vi "Run.vi"(8 "error in (no error)":errorcluster, 11 "Opctics in":refnum<class "Optics.lvclass">) -> (0 "error out":errorcluster, 3 "Optics out":refnum<class "Optics.lvclass">)   [LabVIEW 2018, in "Optics.lvclass"]
uses:
  Optics.lvclass
  Optics.lvclass/Optics.ctl
  Device.lvclass
  StateMachine/State Machine.lvclass
panel:
  out "on target 3":bool
  out "on target 2":bool
  out "on target":bool
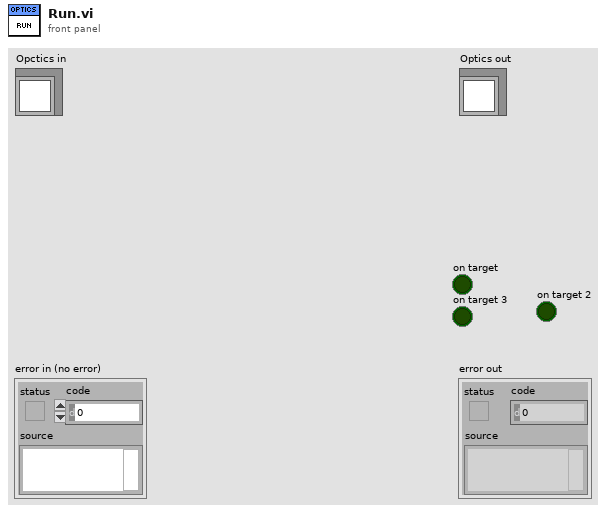
[diagram p1: front panel]
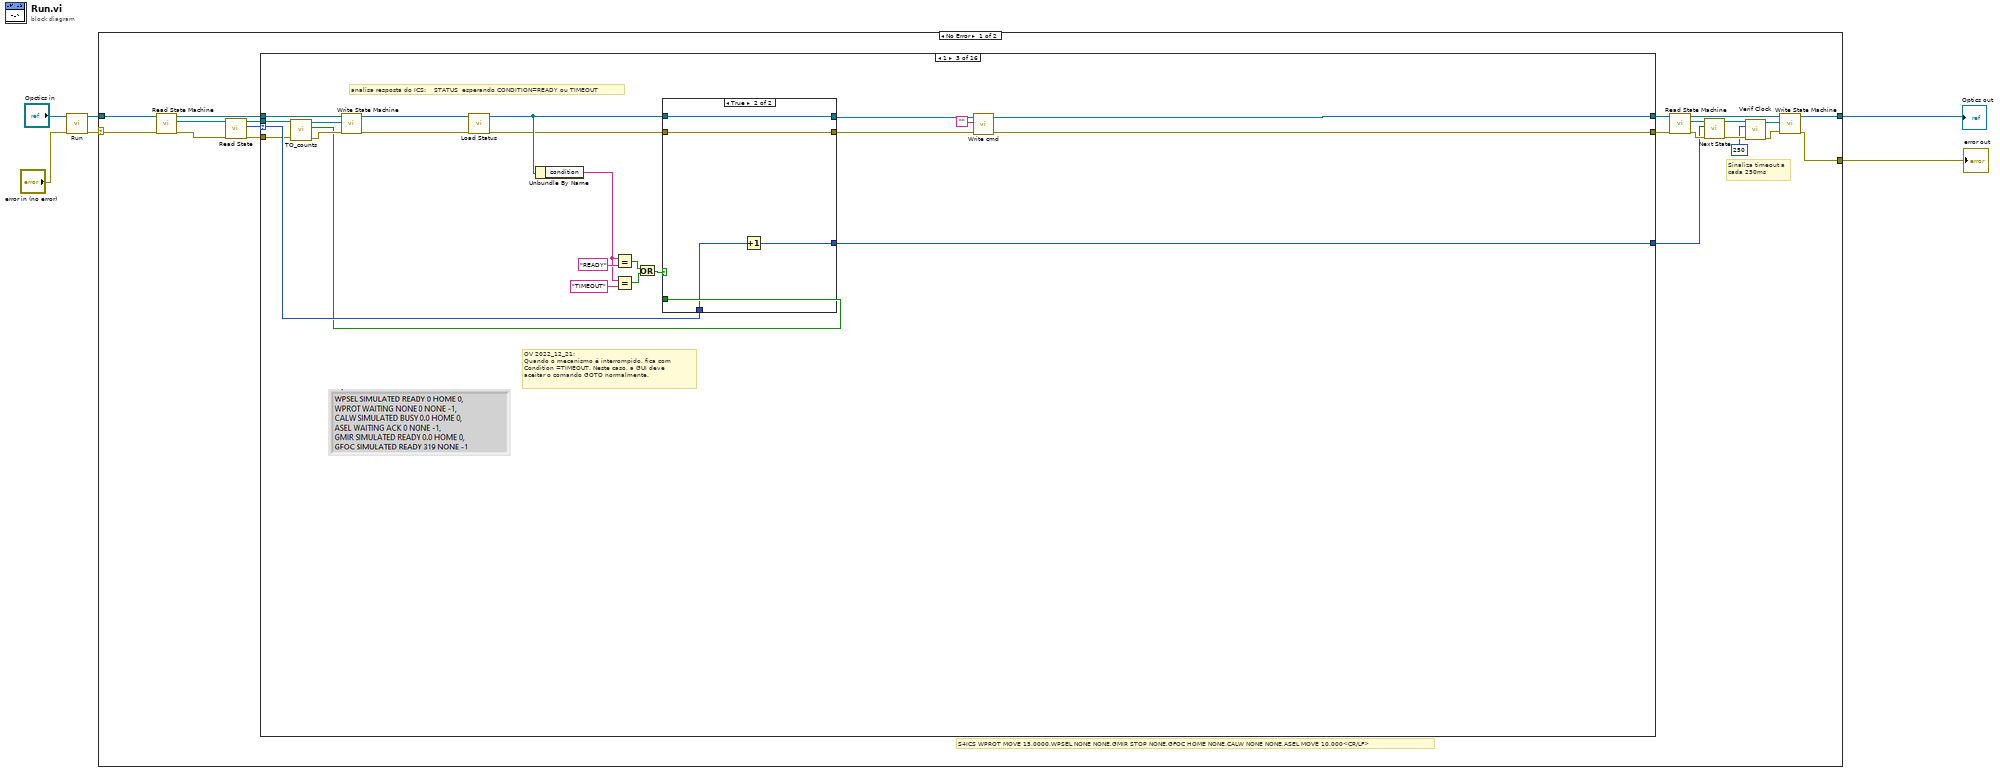
[diagram p0: block diagram]
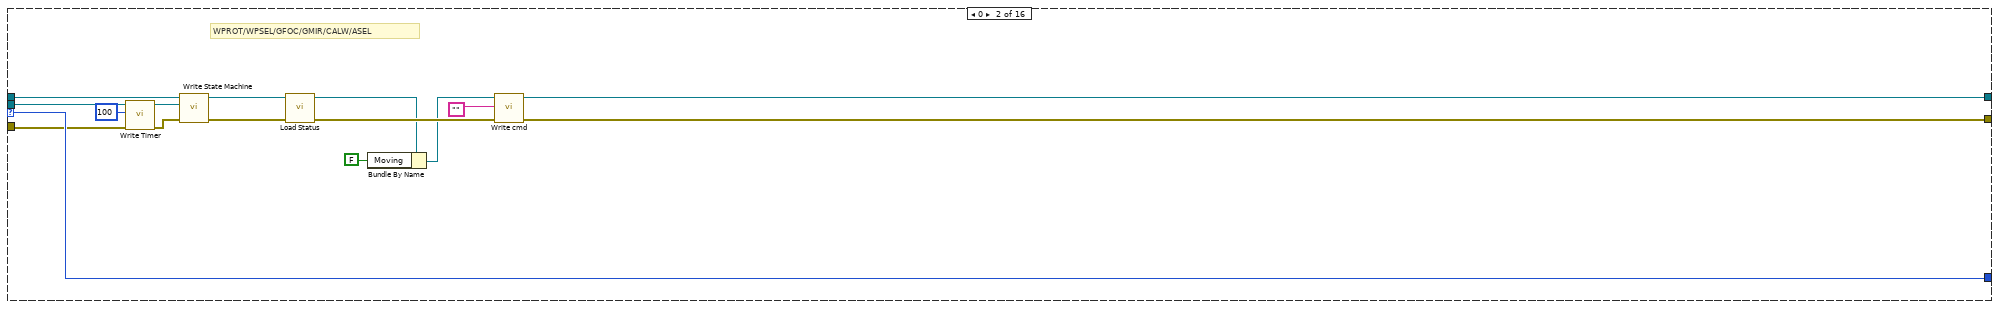
[diagram p3: hidden frame]
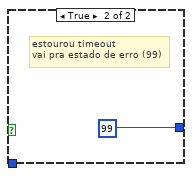
[diagram p5: hidden frame]
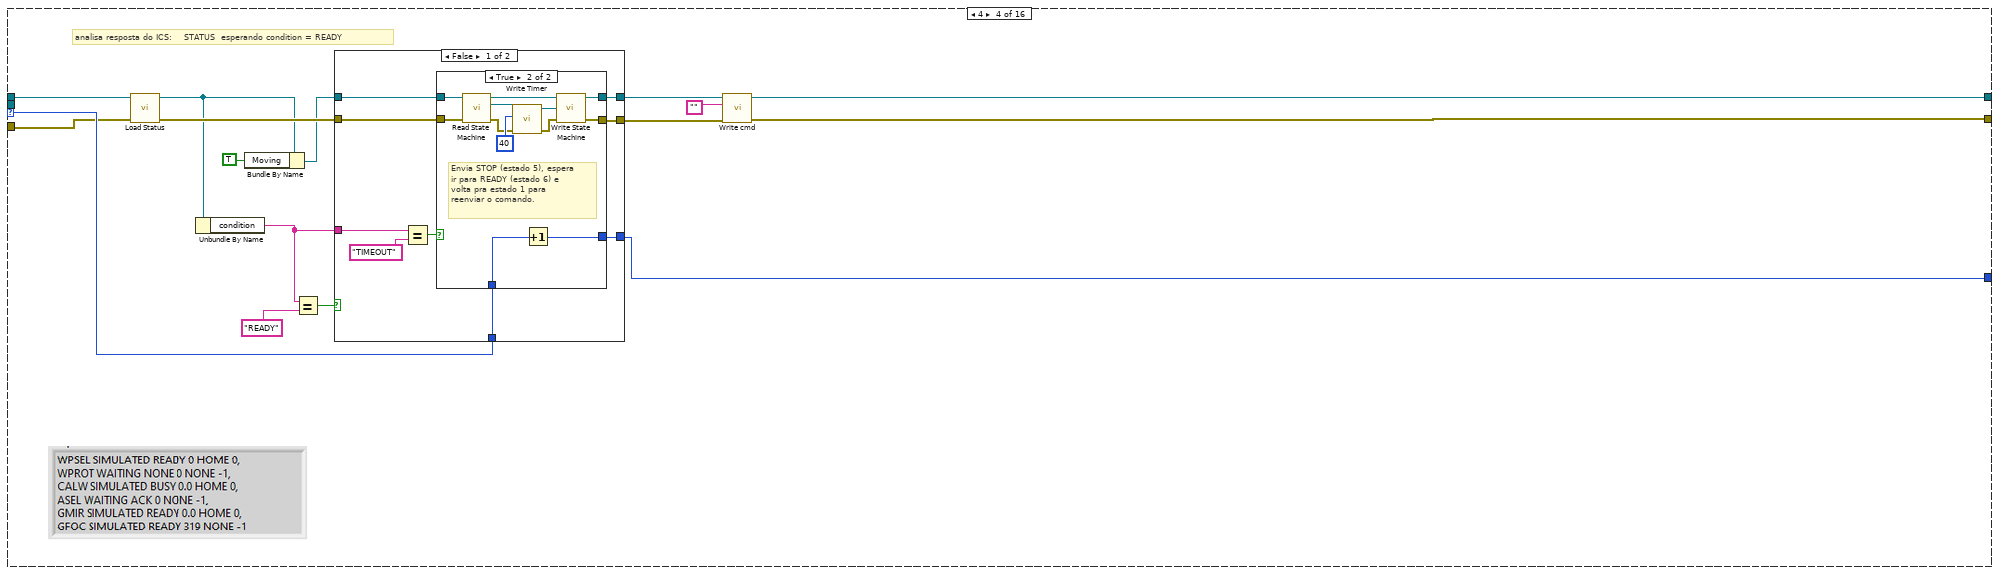
[diagram p6: hidden frame]
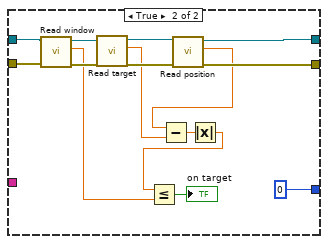
[diagram p8: hidden frame]
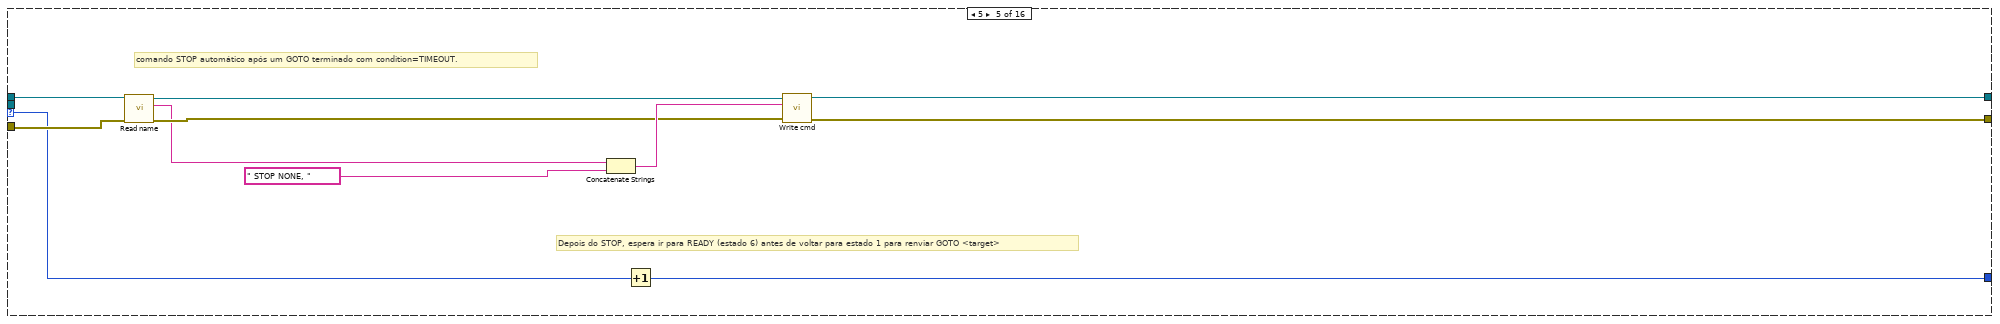
[diagram p9: hidden frame]
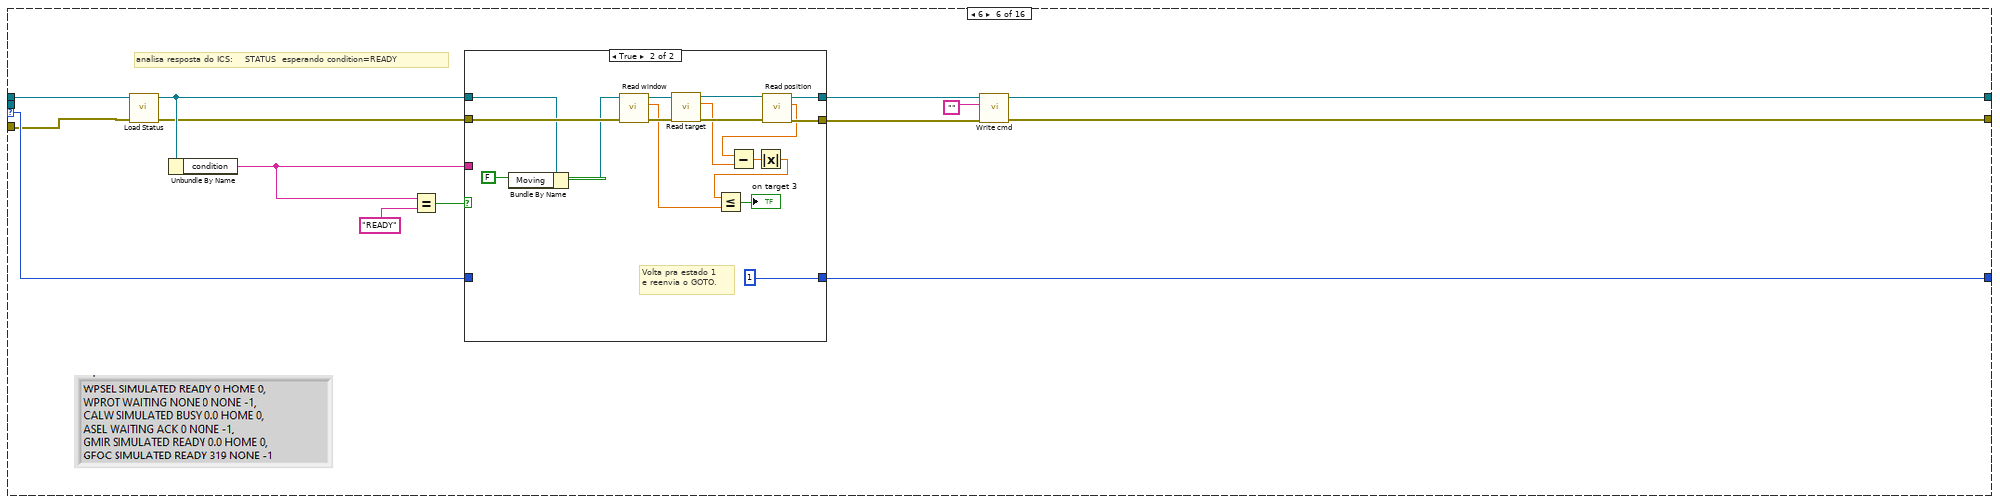
[diagram p10: hidden frame]
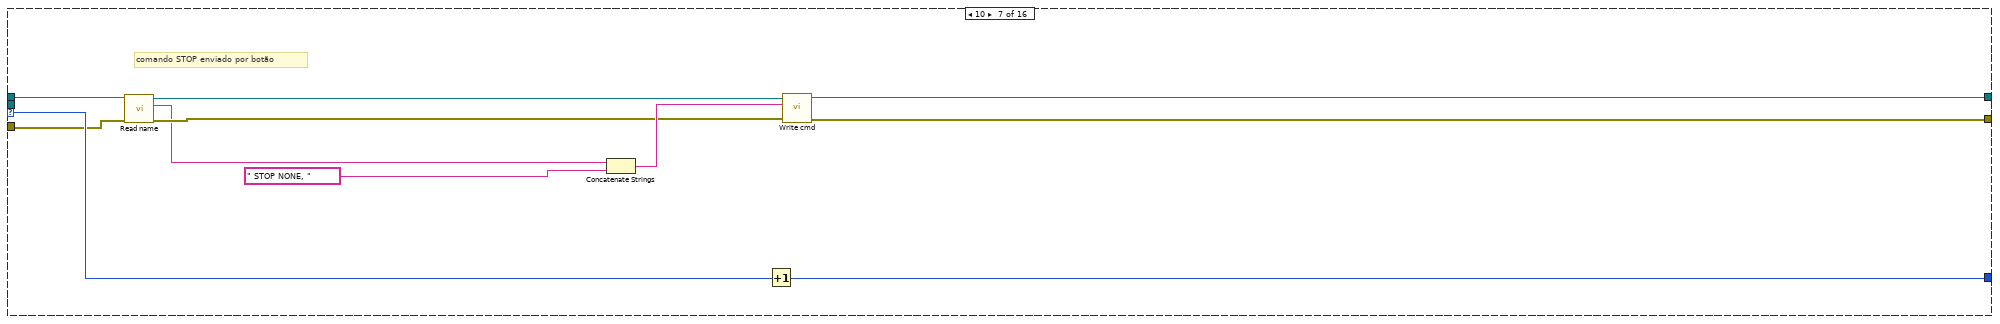
[diagram p12: hidden frame]
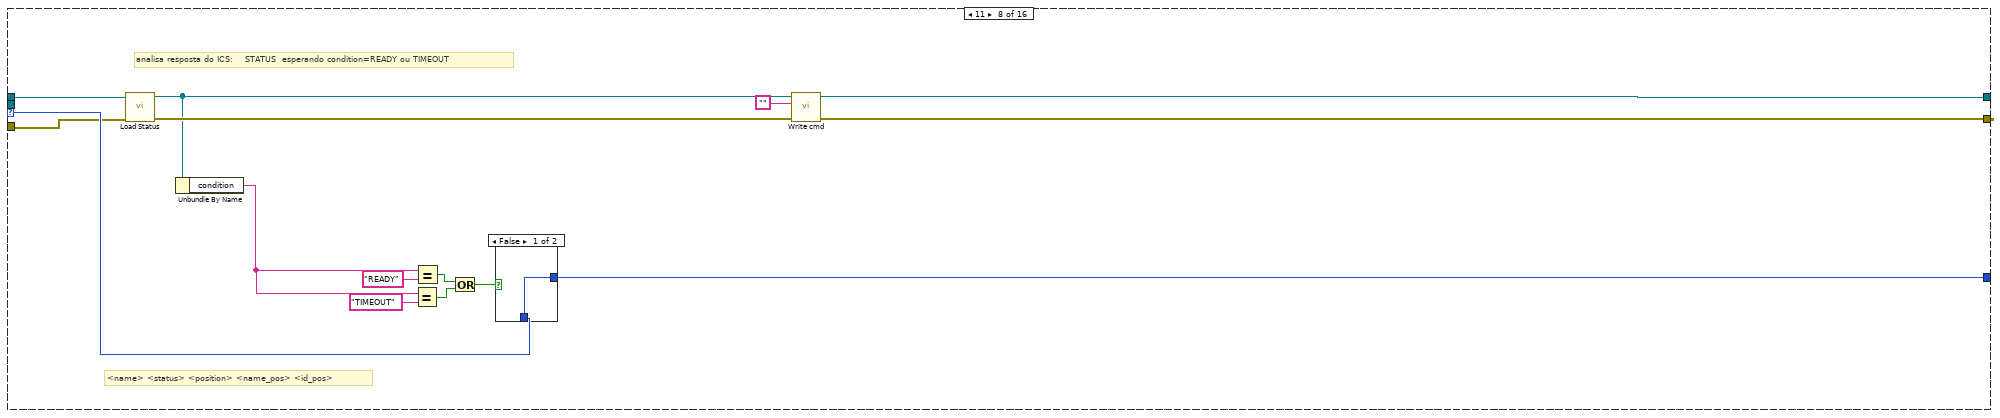
[diagram p13: hidden frame]
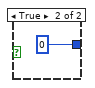
[diagram p14: hidden frame]
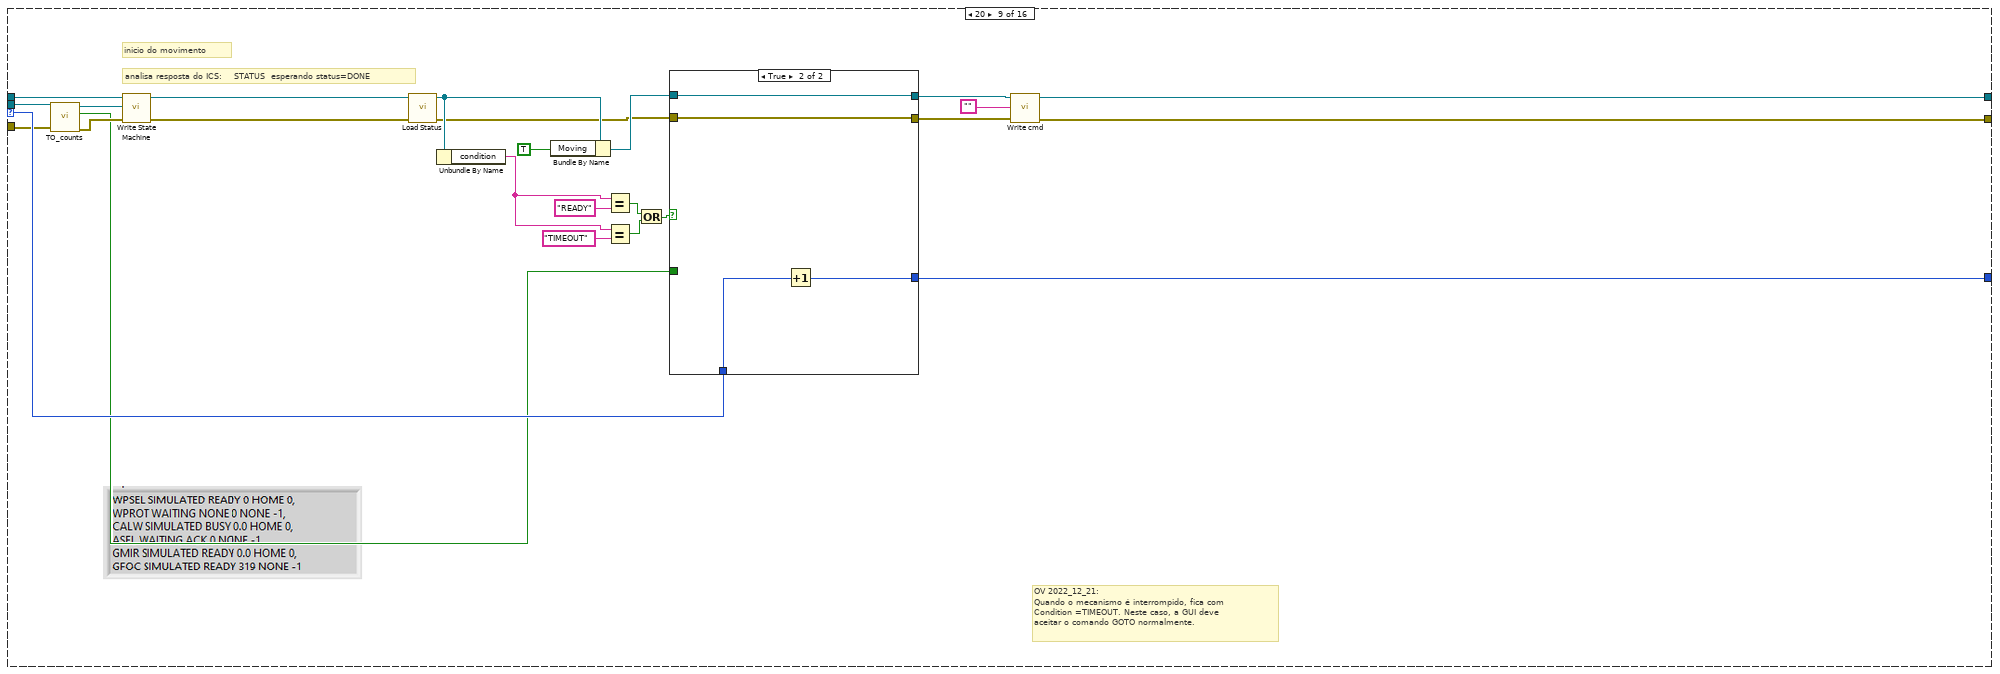
[diagram p15: hidden frame]
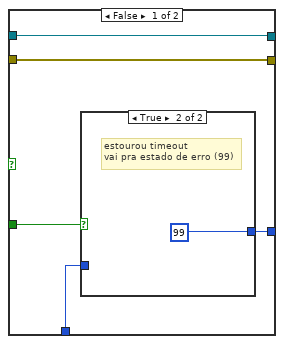
[diagram p16: hidden frame]
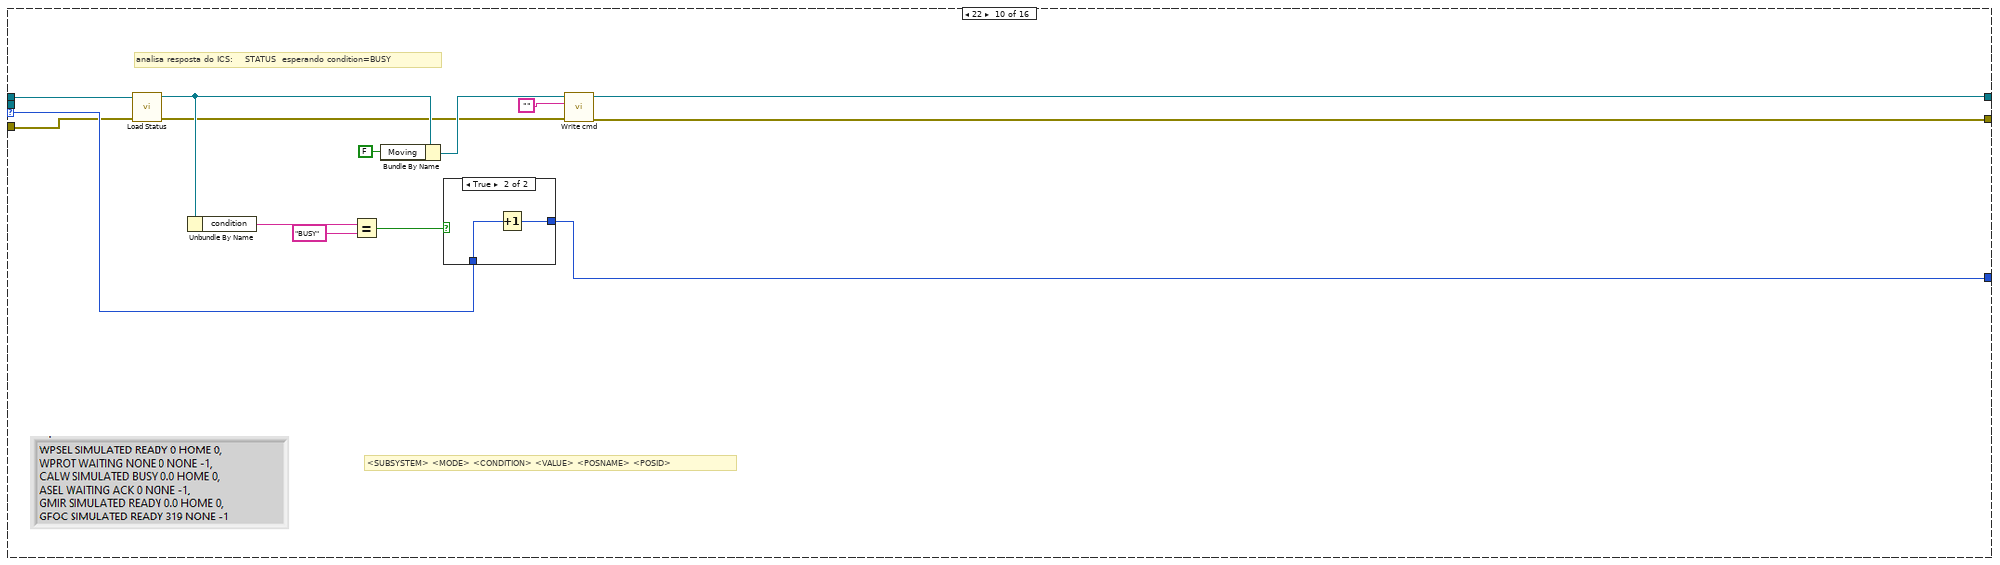
[diagram p18: hidden frame]
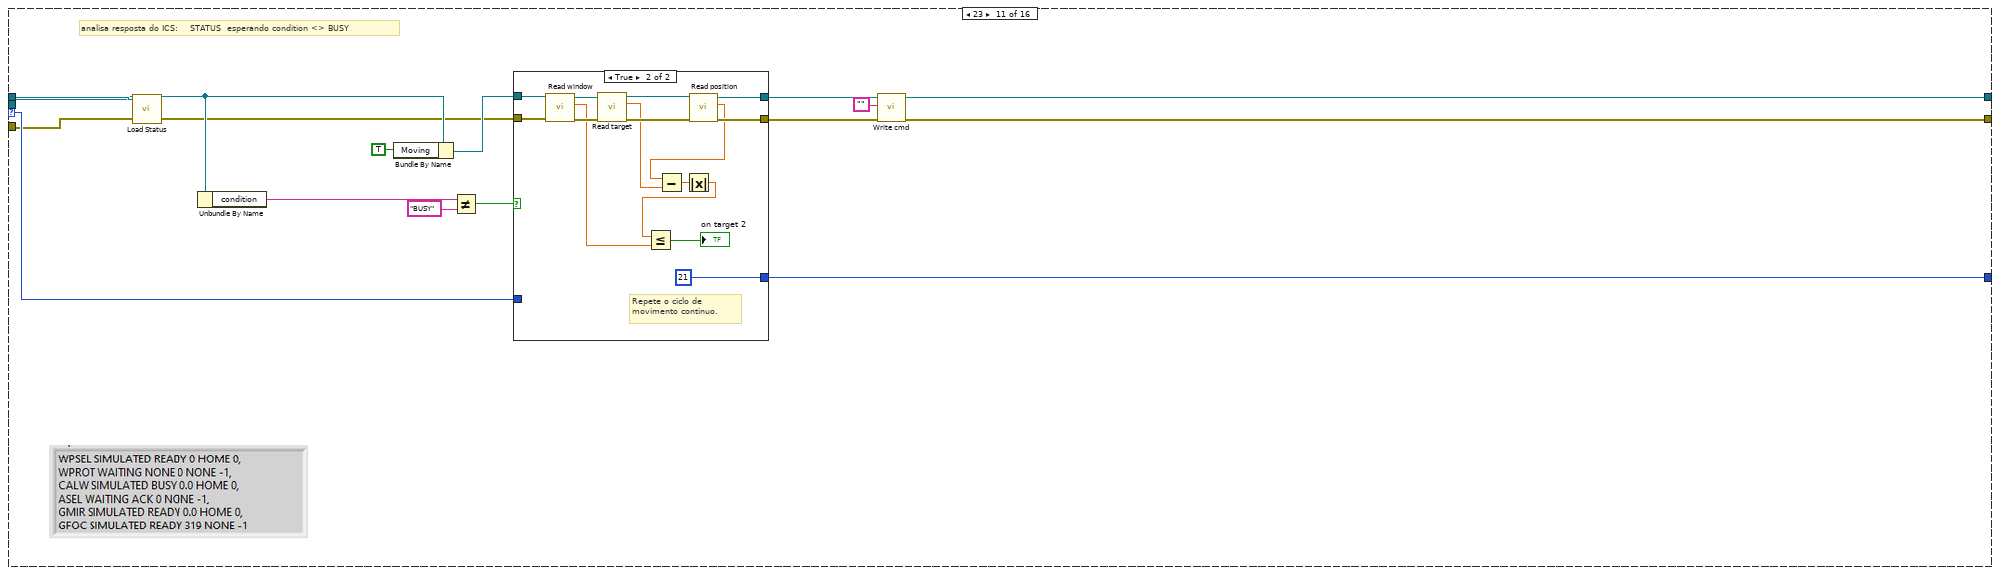
[diagram p20: hidden frame]
diagram:
  n1 = call-parent "Run.vi"("error in (no error)"="error in (no error)", "Device in"="Opctics in") -> ("error out"=w4:errorcluster, "Device out"=w3:refnum<class "Optics.lvclass">)  [unwired: 8 in]
  n2 = case shown="No Error" w4 {
    selector: w4 -> [w16 w392]
    tunnel: [w19 w392] -> w1
    tunnel: [w22 w391] -> w2
    tunnel: w3 -> [w17 w391]
    frame No Error {
      # "Sinaliza timeout a\ncada 250ms"
      # "S4ICS WPROT MOVE 15.0000,WPSEL NONE NONE,GMIR STOP NONE,GFOC HOME NONE,CALW NONE NONE,ASEL MOVE 10.000<CR/LF>"
      n3 = call-dynamic "Read State Machine.vi"("error in (no error)"=w16, "Device in"=w17) -> ("error out"=w15:errorcluster, "State Machine.lvclass"=w14:refnum<class "State Machine.lvclass">, "Device out"=w25:refnum<class "Optics.lvclass">)  [unwired: 7 in]
      n4 = call-dynamic "Read State.vi"("error in (no error)"=w15, "State Machine in"=w14) -> ("error out"=w26:errorcluster, "State"=w27:i32, "State Machine out"=w18:refnum<class "State Machine.lvclass">)  [unwired: 7 in]
      n5 = case shown="1" w27 {
        selector: w27 -> [w28 w43 w66 w93 w137 w157 w188 w206 w230 w258 w274 w308 w330 w349 w368 w388]
        tunnel: w26 -> [w29 w41 w62 w86 w140 w151 w183 w195 w226 w249 w267 w302 w322 w343 w361 w383]
        tunnel: [w29 w45 w68 w95 w145 w159 w190 w203 w232 w255 w276 w311 w327 w347 w365 w389] -> w8
        tunnel: w25 -> [w30 w42 w65 w87 w142 w150 w185 w196 w229 w250 w266 w301 w326 w350 w364 w384]
        tunnel: [w30 w46 w69 w96 w146 w160 w191 w204 w233 w256 w277 w312 w328 w348 w366 w390] -> w7
        tunnel: [w28 w43 w67 w94 w136 w158 w189 w205 w231 w257 w275 w309 w329 w346 w367 w388] -> w20
        tunnel: w18 -> [_ w39 w64 _ _ _ _ _ w228 _ _ w303 w324 w345 w363 _]
        frame Default {
        }
        frame 0 {
          # "WPROT/WPSEL/GFOC/GMIR/CALW/ASEL"
          n6 = call-dynamic "Write Timer.vi"("error in (no error)"=w41, "Timer"=u32 100, "State Machine in"=w39) -> ("error out"=w40:errorcluster, "State Machine out"=w38:refnum<class "State Machine.lvclass">)  [unwired: 7 in]
          n7 = call-dynamic "Write State Machine.vi"("error in (no error)"=w40, "State Machine.lvclass"=w38, "Device in"=w42) -> ("error out"=w35:errorcluster, "Device out"=w36:refnum<class "Optics.lvclass">)  [unwired: 7 in]
          n8 = call-dynamic "Load Status.vi"("error in (no error)"=w35, "Optics in"=w36) -> ("error out"=w34:errorcluster, "Optics out"=w33:refnum<class "Optics.lvclass">)  [unwired: 8 in]
          n9 = Bundle By Name(cluster=w33, "Moving"=FALSE) -> (w31:refnum<class "Optics.lvclass">)
          n10 = call-dynamic "Write cmd.vi"("error in (no error)"=w34, "cmd"="", "Device in"=w31) -> ("error out"=w45:errorcluster, "Device out"=w46:refnum<class "Optics.lvclass">)  [unwired: 7 in]
        }
        frame 1 {
          # "OV 2022_12_21:\nQuando o mecanismo é interrompido, fica com\nCondition =TIMEOUT. Neste caso, a GUI deve\naceitar o comando GOTO normalmente."
          # "analisa resposta do ICS:    STATUS  esperando CONDITION=READY ou TIMEOUT"
          n11 = call-dynamic "TO_counts.vi"("error in (no error)"=w62, "State Machine in"=w64) -> ("error out"=w61:errorcluster, "timer zero"=w60:bool, "State Machine out"=w63:refnum<class "State Machine.lvclass">)  [unwired: 7 in]
          n12 = call-dynamic "Write State Machine.vi"("error in (no error)"=w61, "State Machine.lvclass"=w63, "Device in"=w65) -> ("error out"=w50:errorcluster, "Device out"=w51:refnum<class "Optics.lvclass">)  [unwired: 7 in]
          n13 = call-dynamic "Load Status.vi"("error in (no error)"=w50, "Optics in"=w51) -> ("error out"=w48:errorcluster, "Optics out"=w49:refnum<class "Optics.lvclass">)  [unwired: 8 in]
          n14 = Unbundle By Name(w49) -> ("condition"=w47:string)
          n15 = Equal?(x=w47, y="READY") -> (x = y?=w53:bool)
          n16 = Equal?(x=w47, y="TIMEOUT") -> (x = y?=w52:bool)
          n17 = Or(x=w53, y=w52) -> (x .or. y?=w54:bool)
          n18 = case shown="True" w54 {
            tunnel: [w72 w77] -> w67
            tunnel: w66 -> [w71 w78]
            tunnel: w49 -> [w74 w80]
            tunnel: w48 -> [w73 w79]
            tunnel: [w74 w80] -> w58
            tunnel: [w73 w79] -> w59
            tunnel: w60 -> [w70 _]
            frame False {
              n19 = case shown="False" w70 {
                tunnel: [w75 99 ("State")] -> w72
                tunnel: w71 -> [w75 _]
                frame False {
                  # "Não estourou timeout"
                }
                frame True {
                  # "estourou timeout\nvai pra estado de erro (99)"
                }
              }
            }
            frame True {
              n20 = Increment(x=w78) -> (x+1=w77:i32)
            }
          }
          n21 = call-dynamic "Write cmd.vi"("error in (no error)"=w59, "cmd"="", "Device in"=w58) -> ("error out"=w68:errorcluster, "Device out"=w69:refnum<class "Optics.lvclass">)  [unwired: 7 in]
        }
        frame 4 {
          # "analisa resposta do ICS:    STATUS  esperando condition = READY"
          n22 = call-dynamic "Load Status.vi"("error in (no error)"=w86, "Optics in"=w87) -> ("error out"=w85:errorcluster, "Optics out"=w83:refnum<class "Optics.lvclass">)  [unwired: 8 in]
          n23 = Unbundle By Name(w83) -> ("condition"=w84:string)
          n24 = Bundle By Name(cluster=w83, "Moving"=TRUE) -> (w82:refnum<class "Optics.lvclass">)
          n25 = Equal?(x=w84, y="READY") -> (x = y?=w88:bool)
          n26 = case shown="False" w88 {
            tunnel: [w104 0 ("t")] -> w94
            tunnel: w93 -> [w105 _]
            tunnel: w82 -> [w100 w127]
            tunnel: w85 -> [w98 w125]
            tunnel: [w99 w133] -> w91
            tunnel: [w97 w132] -> w92
            tunnel: w84 -> [w101 _]
            frame False {
              n27 = Equal?(x=w101, y="TIMEOUT") -> (x = y?=w102:bool)
              n28 = case shown="True" w102 {
                tunnel: w105 -> [w108 w110]
                tunnel: [w108 w109] -> w104
                tunnel: w100 -> [w107 w120]
                tunnel: [w107 w115] -> w99
                tunnel: w98 -> [w106 w119]
                tunnel: [w106 w113] -> w97
                frame False {
                }
                frame True {
                  # "Envia STOP (estado 5), espera\nir para READY (estado 6) e\nvolta pra estado 1 para\nreenviar o comando."
                  n29 = call-dynamic "Read State Machine.vi"("error in (no error)"=w119, "Device in"=w120) -> ("error out"=w116:errorcluster, "State Machine.lvclass"=w118:refnum<class "State Machine.lvclass">, "Device out"=w111:refnum<class "Optics.lvclass">)  [unwired: 7 in]
                  n30 = call-dynamic "Write Timer.vi"("error in (no error)"=w116, "Timer"=u32 40, "State Machine in"=w118) -> ("error out"=w114:errorcluster, "State Machine out"=w112:refnum<class "State Machine.lvclass">)  [unwired: 7 in]
                  n31 = Increment(x=w110) -> (x+1=w109:i32)
                  n32 = call-dynamic "Write State Machine.vi"("error in (no error)"=w114, "State Machine.lvclass"=w112, "Device in"=w111) -> ("error out"=w113:errorcluster, "Device out"=w115:refnum<class "Optics.lvclass">)  [unwired: 7 in]
                }
              }
            }
            frame True {
              n33 = call "Read window.vi"("error in (no error)"=w125, "Optics in"=w127) -> ("error out"=w124:errorcluster, "window"=w123:dbl, "Optics out"=w126:refnum<class "Optics.lvclass">)  [unwired: 7 in]
              n34 = call "Read target.vi"("error in (no error)"=w124, "Optics in"=w126) -> ("error out"=w135:errorcluster, "target"=w131:dbl, "Optics out"=w134:refnum<class "Optics.lvclass">)  [unwired: 7 in]
              n35 = call "Read position.vi"("error in (no error)"=w135, "Optics in"=w134) -> ("error out"=w132:errorcluster, "position"=w130:dbl, "Optics out"=w133:refnum<class "Optics.lvclass">)  [unwired: 7 in]
              n36 = Subtract(x=w130, y=w131) -> (x-y=w129:dbl)
              n37 = Absolute Value(x=w129) -> (abs(x)=w128:dbl)
              n38 = Less Or Equal?(x=w128, y=w123) -> (x <= y?=→"on target":bool)
            }
          }
          n39 = call-dynamic "Write cmd.vi"("error in (no error)"=w92, "cmd"="", "Device in"=w91) -> ("error out"=w95:errorcluster, "Device out"=w96:refnum<class "Optics.lvclass">)  [unwired: 7 in]
        }
        frame 5 {
          # "Depois do STOP, espera ir para READY (estado 6) antes de voltar para estado 1 para renviar GOTO <target>"
          # "comando STOP automático após um GOTO terminado com condition=TIMEOUT."
          n40 = call "Read name.vi"("error in (no error)"=w140, "Optics in"=w142) -> ("error out"=w139:errorcluster, "name"=w138:string, "Optics out"=w141:refnum<class "Optics.lvclass">)  [unwired: 7 in]
          n41 = Concatenate Strings(w138, " STOP NONE, " ("string")) -> (w143:string)
          n42 = Increment(x=w137) -> (x+1=w136:i32)
          n43 = call-dynamic "Write cmd.vi"("error in (no error)"=w139, "cmd"=w143, "Device in"=w141) -> ("error out"=w145:errorcluster, "Device out"=w146:refnum<class "Optics.lvclass">)  [unwired: 7 in]
        }
        frame 6 {
          # "analisa resposta do ICS:    STATUS  esperando condition=READY"
          n44 = call-dynamic "Load Status.vi"("error in (no error)"=w151, "Optics in"=w150) -> ("error out"=w147:errorcluster, "Optics out"=w148:refnum<class "Optics.lvclass">)  [unwired: 8 in]
          n45 = Unbundle By Name(w148) -> ("condition"=w149:string)
          n46 = Equal?(x=w149, y="READY") -> (x = y?=w152:bool)
          n47 = case shown="True" w152 {
            tunnel: [w163 1 ("t")] -> w158
            tunnel: w157 -> [w163 _]
            tunnel: w148 -> [w161 w165]
            tunnel: w147 -> [w162 w171]
            tunnel: [w161 w178] -> w155
            tunnel: [w162 w177] -> w156
            tunnel: w149 -> [_ _]
            frame False {
            }
            frame True {
              # "Volta pra estado 1 \ne reenvia o GOTO."
              n48 = Bundle By Name(cluster=w165, "Moving"=FALSE) -> (w164:refnum<class "Optics.lvclass">)
              n49 = call "Read window.vi"("error in (no error)"=w171, "Optics in"=w164) -> ("error out"=w170:errorcluster, "window"=w169:dbl, "Optics out"=w172:refnum<class "Optics.lvclass">)  [unwired: 7 in]
              n50 = call "Read target.vi"("error in (no error)"=w170, "Optics in"=w172) -> ("error out"=w180:errorcluster, "target"=w176:dbl, "Optics out"=w179:refnum<class "Optics.lvclass">)  [unwired: 7 in]
              n51 = call "Read position.vi"("error in (no error)"=w180, "Optics in"=w179) -> ("error out"=w177:errorcluster, "position"=w175:dbl, "Optics out"=w178:refnum<class "Optics.lvclass">)  [unwired: 7 in]
              n52 = Subtract(x=w175, y=w176) -> (x-y=w174:dbl)
              n53 = Absolute Value(x=w174) -> (abs(x)=w173:dbl)
              n54 = Less Or Equal?(x=w173, y=w169) -> (x <= y?=→"on target 3":bool)
            }
          }
          n55 = call-dynamic "Write cmd.vi"("error in (no error)"=w156, "cmd"="", "Device in"=w155) -> ("error out"=w159:errorcluster, "Device out"=w160:refnum<class "Optics.lvclass">)  [unwired: 7 in]
        }
        frame 10 {
          # "comando STOP enviado por botão"
          n56 = call "Read name.vi"("error in (no error)"=w183, "Optics in"=w185) -> ("error out"=w182:errorcluster, "name"=w181:string, "Optics out"=w184:refnum<class "Optics.lvclass">)  [unwired: 7 in]
          n57 = Concatenate Strings(w181, " STOP NONE, " ("string")) -> (w186:string)
          n58 = Increment(x=w188) -> (x+1=w189:i32)
          n59 = call-dynamic "Write cmd.vi"("error in (no error)"=w182, "cmd"=w186, "Device in"=w184) -> ("error out"=w190:errorcluster, "Device out"=w191:refnum<class "Optics.lvclass">)  [unwired: 7 in]
        }
        frame 11 {
          # "<name> <status> <position> <name_pos> <id_pos>"
          # "analisa resposta do ICS:    STATUS  esperando condition=READY ou TIMEOUT"
          n60 = call-dynamic "Load Status.vi"("error in (no error)"=w195, "Optics in"=w196) -> ("error out"=w193:errorcluster, "Optics out"=w192:refnum<class "Optics.lvclass">)  [unwired: 8 in]
          n61 = Unbundle By Name(w192) -> ("condition"=w194:string)
          n62 = Equal?(x=w194, y="TIMEOUT") -> (x = y?=w198:bool)
          n63 = Equal?(x=w194, y="READY") -> (x = y?=w199:bool)
          n64 = Or(x=w199, y=w198) -> (x .or. y?=w197:bool)
          n65 = case shown="False" w197 {
            tunnel: [w207 0] -> w205
            tunnel: w206 -> [w207 _]
            frame False {
            }
            frame True {
            }
          }
          n66 = call-dynamic "Write cmd.vi"("error in (no error)"=w193, "cmd"="", "Device in"=w192) -> ("error out"=w203:errorcluster, "Device out"=w204:refnum<class "Optics.lvclass">)  [unwired: 7 in]
        }
        frame 20 {
          # "OV 2022_12_21:\nQuando o mecanismo é interrompido, fica com\nCondition =TIMEOUT. Neste caso, a GUI deve\naceitar o comando GOTO normalmente."
          # "inicio do movimento"
          # "analisa resposta do ICS:    STATUS  esperando status=DONE"
          n67 = call-dynamic "TO_counts.vi"("error in (no error)"=w226, "State Machine in"=w228) -> ("error out"=w225:errorcluster, "timer zero"=w224:bool, "State Machine out"=w227:refnum<class "State Machine.lvclass">)  [unwired: 7 in]
          n68 = call-dynamic "Write State Machine.vi"("error in (no error)"=w225, "State Machine.lvclass"=w227, "Device in"=w229) -> ("error out"=w213:errorcluster, "Device out"=w214:refnum<class "Optics.lvclass">)  [unwired: 7 in]
          n69 = call-dynamic "Load Status.vi"("error in (no error)"=w213, "Optics in"=w214) -> ("error out"=w209:errorcluster, "Optics out"=w211:refnum<class "Optics.lvclass">)  [unwired: 8 in]
          n70 = Unbundle By Name(w211) -> ("condition"=w212:string)
          n71 = Bundle By Name(cluster=w211, "Moving"=TRUE) -> (w210:refnum<class "Optics.lvclass">)
          n72 = Equal?(x=w212, y="READY") -> (x = y?=w216:bool)
          n73 = Equal?(x=w212, y="TIMEOUT") -> (x = y?=w215:bool)
          n74 = Or(x=w216, y=w215) -> (x .or. y?=w217:bool)
          n75 = case shown="True" w217 {
            tunnel: [w236 w241] -> w231
            tunnel: w230 -> [w235 w242]
            tunnel: w210 -> [w238 w244]
            tunnel: w209 -> [w237 w243]
            tunnel: [w238 w244] -> w221
            tunnel: [w237 w243] -> w222
            tunnel: w224 -> [w234 _]
            frame False {
              n76 = case shown="True" w234 {
                tunnel: [w239 99 ("State")] -> w236
                tunnel: w235 -> [w239 _]
                frame False {
                  # "Não estourou timeout"
                }
                frame True {
                  # "estourou timeout\nvai pra estado de erro (99)"
                }
              }
            }
            frame True {
              n77 = Increment(x=w242) -> (x+1=w241:i32)
            }
          }
          n78 = call-dynamic "Write cmd.vi"("error in (no error)"=w222, "cmd"="", "Device in"=w221) -> ("error out"=w232:errorcluster, "Device out"=w233:refnum<class "Optics.lvclass">)  [unwired: 7 in]
        }
        frame 22 {
          # "<SUBSYSTEM> <MODE> <CONDITION> <VALUE> <POSNAME> <POSID>"
          # "analisa resposta do ICS:    STATUS  esperando condition=BUSY"
          n79 = call-dynamic "Load Status.vi"("error in (no error)"=w249, "Optics in"=w250) -> ("error out"=w245:errorcluster, "Optics out"=w247:refnum<class "Optics.lvclass">)  [unwired: 8 in]
          n80 = Unbundle By Name(w247) -> ("condition"=w248:string)
          n81 = Equal?(x=w248, y="BUSY") -> (x = y?=w251:bool)
          n82 = Bundle By Name(cluster=w247, "Moving"=FALSE) -> (w246:refnum<class "Optics.lvclass">)
          n83 = case shown="True" w251 {
            tunnel: [w259 w260] -> w257
            tunnel: w258 -> [w259 w261]
            frame False {
            }
            frame True {
              n84 = Increment(x=w261) -> (x+1=w260:i32)
            }
          }
          n85 = call-dynamic "Write cmd.vi"("error in (no error)"=w245, "cmd"="", "Device in"=w246) -> ("error out"=w255:errorcluster, "Device out"=w256:refnum<class "Optics.lvclass">)  [unwired: 7 in]
        }
        frame 23 {
          # "analisa resposta do ICS:    STATUS  esperando condition <> BUSY"
          n86 = call-dynamic "Load Status.vi"("error in (no error)"=w267, "Optics in"=w266) -> ("error out"=w262:errorcluster, "Optics out"=w264:refnum<class "Optics.lvclass">)  [unwired: 8 in]
          n87 = Unbundle By Name(w264) -> ("condition"=w265:string)
          n88 = Bundle By Name(cluster=w264, "Moving"=TRUE) -> (w263:refnum<class "Optics.lvclass">)
          n89 = Not Equal?(x=w265, y="BUSY") -> (x != y?=w269:bool)
          n90 = case shown="True" w269 {
            tunnel: [w280 21 ("t")] -> w275
            tunnel: w274 -> [w280 _]
            tunnel: w263 -> [w279 w287]
            tunnel: w262 -> [w278 w285]
            tunnel: [w279 w293] -> w272
            tunnel: [w278 w292] -> w271
            frame False {
            }
            frame True {
              # "Repete o ciclo de\nmovimento continuo."
              n91 = call "Read window.vi"("error in (no error)"=w285, "Optics in"=w287) -> ("error out"=w284:errorcluster, "window"=w283:dbl, "Optics out"=w286:refnum<class "Optics.lvclass">)  [unwired: 7 in]
              n92 = call "Read target.vi"("error in (no error)"=w284, "Optics in"=w286) -> ("error out"=w295:errorcluster, "target"=w291:dbl, "Optics out"=w294:refnum<class "Optics.lvclass">)  [unwired: 7 in]
              n93 = call "Read position.vi"("error in (no error)"=w295, "Optics in"=w294) -> ("error out"=w292:errorcluster, "position"=w290:dbl, "Optics out"=w293:refnum<class "Optics.lvclass">)  [unwired: 7 in]
              n94 = Subtract(x=w290, y=w291) -> (x-y=w289:dbl)
              n95 = Absolute Value(x=w289) -> (abs(x)=w288:dbl)
              n96 = Less Or Equal?(x=w288, y=w283) -> (x <= y?=→"on target 2":bool)
            }
          }
          n97 = call-dynamic "Write cmd.vi"("error in (no error)"=w271, "cmd"="", "Device in"=w272) -> ("error out"=w276:errorcluster, "Device out"=w277:refnum<class "Optics.lvclass">)  [unwired: 7 in]
        }
        frame 30 {
          # "240 x 0,25s = 1min \npara completar homing"
          # "S4ICS GMIR INIT NONE"
          # "WPROT/WPSEL/GFOC/GMIR/CALW/ASEL"
          # "comando INIT"
          n98 = call-dynamic "Write Timer.vi"("error in (no error)"=w302, "Timer"=u32 240, "State Machine in"=w303) -> ("error out"=w298:errorcluster, "State Machine out"=w297:refnum<class "State Machine.lvclass">)  [unwired: 7 in]
          n99 = call-dynamic "Write State Machine.vi"("error in (no error)"=w298, "State Machine.lvclass"=w297, "Device in"=w301) -> ("error out"=w299:errorcluster, "Device out"=w300:refnum<class "Optics.lvclass">)  [unwired: 7 in]
          n100 = call "Read name.vi"("error in (no error)"=w299, "Optics in"=w300) -> ("error out"=w306:errorcluster, "name"=w304:string, "Optics out"=w305:refnum<class "Optics.lvclass">)  [unwired: 7 in]
          n101 = Concatenate Strings(w304, " INIT NONE, " ("string")) -> (w310:string)
          n102 = Increment(x=w308) -> (x+1=w309:i32)
          n103 = call-dynamic "Write cmd.vi"("error in (no error)"=w306, "cmd"=w310, "Device in"=w305) -> ("error out"=w311:errorcluster, "Device out"=w312:refnum<class "Optics.lvclass">)  [unwired: 7 in]
        }
        frame 31 {
          # "Timeout controlado\npor Verif Clock.vi"
          # "<name> <status> <position> <name_pos> <id_pos>"
          # "analisa resposta do ICS:    STATUS  esperando condition=BUSY"
          n104 = call-dynamic "Read Timeout.vi"("error in (no error)"=w322, "State Machine in"=w324) -> ("error out"=w321:errorcluster, "Timeout"=w320:bool, "State Machine out"=w323:refnum<class "State Machine.lvclass">)  [unwired: 7 in]
          n105 = call-dynamic "Write State Machine.vi"("error in (no error)"=w321, "State Machine.lvclass"=w323, "Device in"=w326) -> ("error out"=w316:errorcluster, "Device out"=w317:refnum<class "Optics.lvclass">)  [unwired: 7 in]
          n106 = call-dynamic "Load Status.vi"("error in (no error)"=w316, "Optics in"=w317) -> ("error out"=w314:errorcluster, "Optics out"=w313:refnum<class "Optics.lvclass">)  [unwired: 8 in]
          n107 = Unbundle By Name(w313) -> ("condition"=w315:string)
          n108 = Equal?(x=w315, y="BUSY") -> (x = y?=w319:bool)
          n109 = case shown="True" w319 {
            tunnel: [w332 w339] -> w329
            tunnel: w330 -> [w333 w340]
            tunnel: w320 -> [w331 _]
            frame False {
              n110 = case shown="True" w331 {
                tunnel: [w334 w336] -> w332
                tunnel: w333 -> [w334 w335]
                frame False {
                }
                frame True {
                  n111 = disable-structure shown="Enabled" {
                    disable-tunnel: [99 ("State") w338] -> w336
                    disable-tunnel: w335 -> [_ w338]
                    frame Disabled {
                    }
                    frame Enabled {
                    }
                  }
                }
              }
            }
            frame True {
              n112 = Increment(x=w340) -> (x+1=w339:i32)
            }
          }
          n113 = call-dynamic "Write cmd.vi"("error in (no error)"=w314, "cmd"="", "Device in"=w313) -> ("error out"=w327:errorcluster, "Device out"=w328:refnum<class "Optics.lvclass">)  [unwired: 7 in]
        }
        frame 32 {
          # "<name> <status> <position> <name_pos> <id_pos>"
          # "timeout  para terminar o movimento: 240 x 0,25s = 1 min"
          n114 = call-dynamic "Write Timer.vi"("error in (no error)"=w343, "Timer"=u32 240, "State Machine in"=w345) -> ("error out"=w342:errorcluster, "State Machine out"=w344:refnum<class "State Machine.lvclass">)  [unwired: 7 in]
          n115 = Increment(x=w349) -> (x+1=w346:i32)
          n116 = call-dynamic "Write State Machine.vi"("error in (no error)"=w342, "State Machine.lvclass"=w344, "Device in"=w350) -> ("error out"=w347:errorcluster, "Device out"=w348:refnum<class "Optics.lvclass">)  [unwired: 7 in]
        }
        frame 33 {
          # "<name> <status> <position> <name_pos> <id_pos>"
          # "analisa resposta do ICS:    STATUS  esperando condition <> BUSY"
          n117 = call-dynamic "TO_counts.vi"("error in (no error)"=w361, "State Machine in"=w363) -> ("error out"=w360:errorcluster, "timer zero"=w359:bool, "State Machine out"=w362:refnum<class "State Machine.lvclass">)  [unwired: 7 in]
          n118 = call-dynamic "Write State Machine.vi"("error in (no error)"=w360, "State Machine.lvclass"=w362, "Device in"=w364) -> ("error out"=w354:errorcluster, "Device out"=w355:refnum<class "Optics.lvclass">)  [unwired: 7 in]
          n119 = call-dynamic "Load Status.vi"("error in (no error)"=w354, "Optics in"=w355) -> ("error out"=w352:errorcluster, "Optics out"=w351:refnum<class "Optics.lvclass">)  [unwired: 8 in]
          n120 = Unbundle By Name(w351) -> ("condition"=w353:string)
          n121 = Not Equal?(x=w353, y="BUSY") -> (x != y?=w356:bool)
          n122 = case shown="True" w356 {
            tunnel: [w370 w380] -> w367
            tunnel: w368 -> [w371 _]
            tunnel: w359 -> [w369 _]
            tunnel: w353 -> [_ w378]
            frame False {
              n123 = case shown="False" w369 {
                tunnel: [w372 w374] -> w370
                tunnel: w371 -> [w372 w373]
                frame False {
                }
                frame True {
                  n124 = disable-structure shown="Disabled" {
                    disable-tunnel: [99 ("State") w376] -> w374
                    disable-tunnel: w373 -> [_ w376]
                    frame Disabled {
                    }
                    frame Enabled {
                    }
                  }
                }
              }
            }
            frame True {
              n125 = Equal?(x="READY" ("y"), y=w378) -> (x = y?=w382:bool)
              n126 = Select(t=0, s=w382, f=30) -> (s? t:f=w380:i32)
            }
          }
          n127 = call-dynamic "Write cmd.vi"("error in (no error)"=w352, "cmd"="", "Device in"=w351) -> ("error out"=w365:errorcluster, "Device out"=w366:refnum<class "Optics.lvclass">)  [unwired: 7 in]
        }
        frame 99 {
          # "WPROT/WPSEL/GFOC/GMIR/CALW/ASEL"
          n128 = call-dynamic "Load Status.vi"("error in (no error)"=w383, "Optics in"=w384) -> ("error out"=w385:errorcluster, "Optics out"=w386:refnum<class "Optics.lvclass">)  [unwired: 8 in]
          n129 = call-dynamic "Write cmd.vi"("error in (no error)"=w385, "cmd"="", "Device in"=w386) -> ("error out"=w389:errorcluster, "Device out"=w390:refnum<class "Optics.lvclass">)  [unwired: 7 in]
        }
      }
      n130 = call-dynamic "Read State Machine.vi"("error in (no error)"=w8, "Device in"=w7) -> ("error out"=w21:errorcluster, "State Machine.lvclass"=w24:refnum<class "State Machine.lvclass">, "Device out"=w23:refnum<class "Optics.lvclass">)  [unwired: 7 in]
      n131 = call "Next State.vi"("error in (no error)"=w21, "New_State"=w20, "State Machine in"=w24) -> ("error out"=w13:errorcluster, "State Machine out"=w11:refnum<class "State Machine.lvclass">)  [unwired: 7 in]
      n132 = call-dynamic "Verif Clock.vi"("error in (no error)"=w13, "period (ms)"=u32 250 ("period"), "State Machine in"=w11) -> ("error out"=w12:errorcluster, "State Machine out"=w10:refnum<class "State Machine.lvclass">)  [unwired: 6 in, 1 out]
      n133 = call-dynamic "Write State Machine.vi"("error in (no error)"=w12, "State Machine.lvclass"=w10, "Device in"=w23) -> ("error out"=w19:errorcluster, "Device out"=w22:refnum<class "Optics.lvclass">)  [unwired: 7 in]
    }
    frame Error {
    }
  }
  "error out" <- w1
  "Optics out" <- w2
